vi "Script Add Constant VI --Project.vi"(4 "Project Ref":refnum<vi>, 6 "App Ref":refnum<vi>, 7 "Constant VI Name":string="TESTING.vi", 8 "error in":errorcluster, 9 "Constant VI Args":refnum<vi>) -> (0 "error out":errorcluster, 3 "Constant VI Path":path)   [LabVIEW 2020, in "ConstantErrorsMaker.lvlib"]
uses:
  ConstantErrorsMaker.lvlib
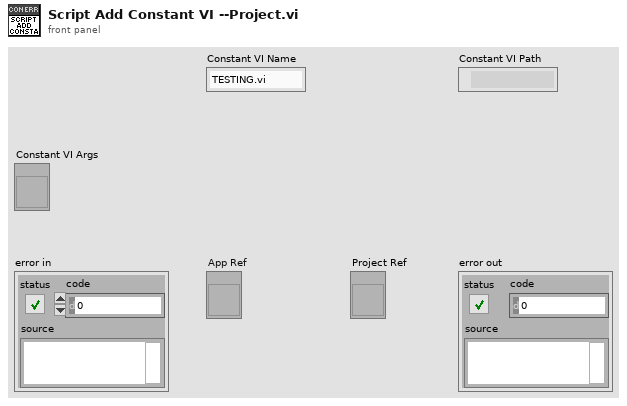
[diagram p1: front panel]
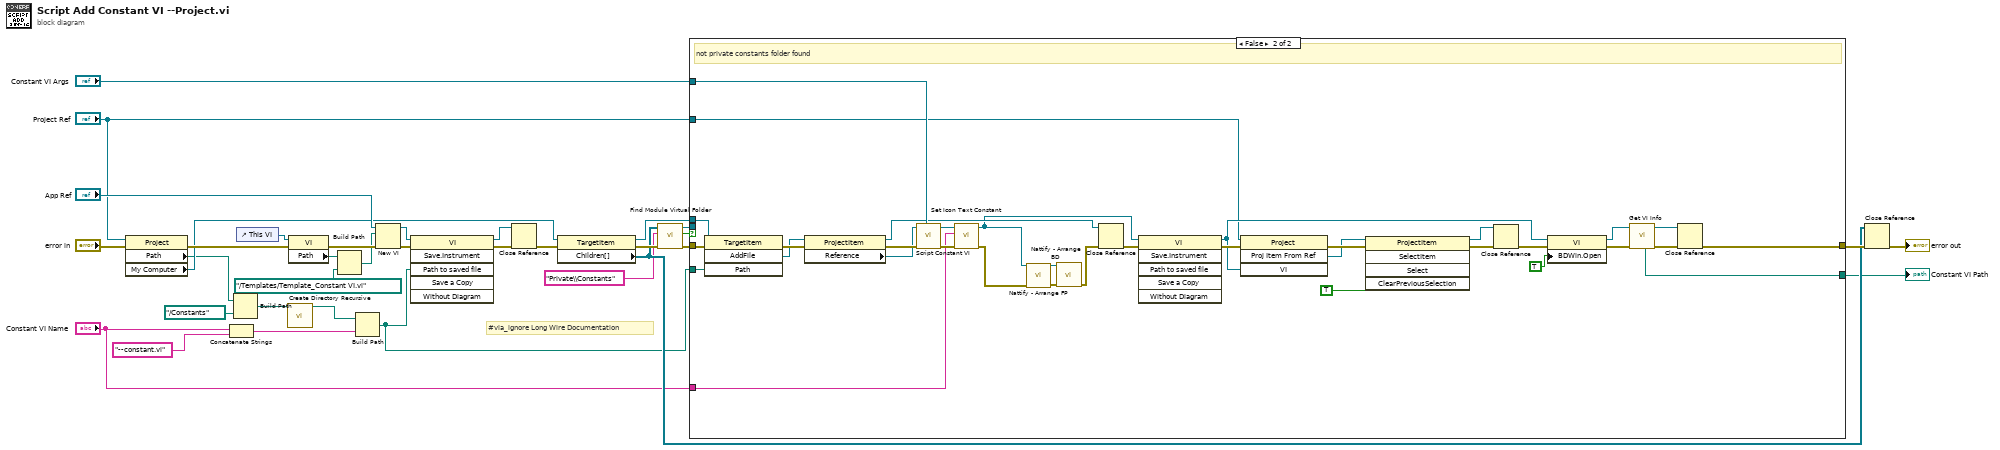
[diagram p0: block diagram]
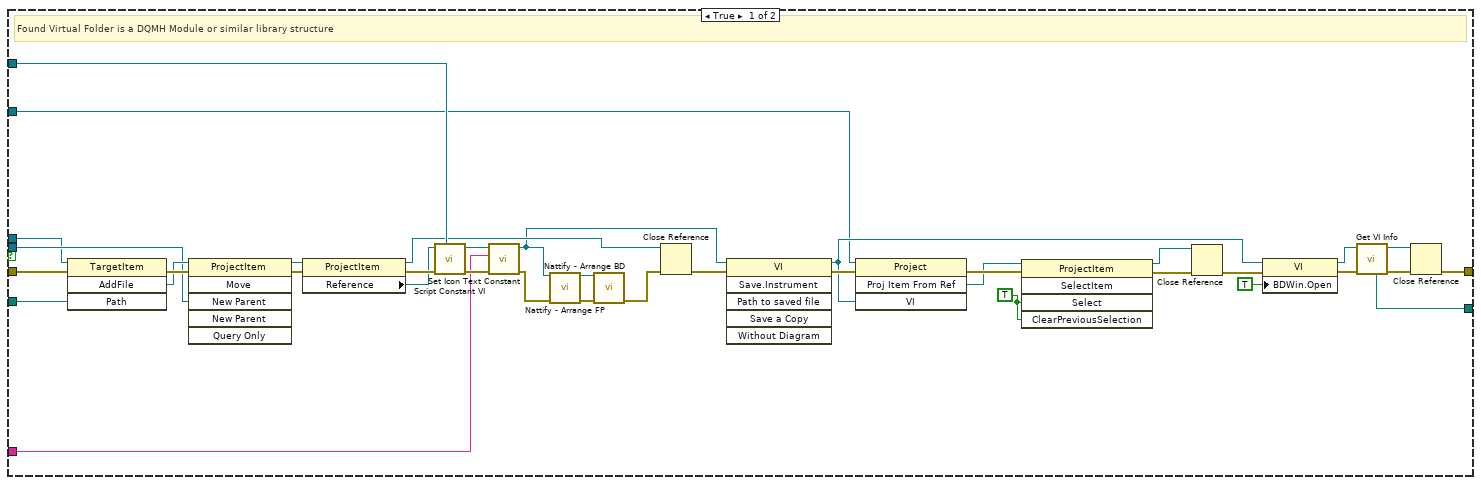
[diagram p2: hidden frame]
diagram:
  # "#via_ignore Long Wire Documentation"
  n1 = property class="Project"(reference="Project Ref", error in="error in") -> (error out=w31:errorcluster, "Path"=w4:path, "My Computer"=w5:refnum<vi>)  [unwired: 1 out]
  n2 = Concatenate Strings("Constant VI Name", "--constant.vi" ("input 1")) -> (w16:string)
  n3 = Build Path(base path=w4, name or relative path=path "../Constants") -> (appended path=w3:path)
  n4 = control-ref of="This VI"() -> (w15:refnum<vi>)
  n5 = call <vilib>:"Create Directory Recursive.vi"("directory"=w3) -> ("directory copy"=w1:path)  [unwired: 4 in, 2 out]
  n6 = property class="VI"(reference=w15, error in=w31) -> (error out=w25:errorcluster, "Path"=w14:path)  [unwired: 1 out]
  n7 = Build Path(base path=w14, name or relative path=path "../Templates/Template_Constant VI.vi") -> (appended path=w13:path)
  n8 = Build Path(base path=w1, name or relative path=w16) -> (appended path=w17:path)
  n9 = New VI(8:w25, 10:w13, 11:"App Ref") -> (0:w28:errorcluster, 3:w19:refnum<vi>)  [unwired: 4 in]
  n10 = invoke class="VI" method="Save.Instrument"(reference=w19, error in=w28, "Path to saved file"=w17) -> (reference out=w11:refnum<vi>, error out=w26:errorcluster)  [unwired: 3 in, 4 out]
  n11 = Close Reference(reference=w11, error in (no error)=w26) -> (error out=w27:errorcluster)
  n12 = property class="TargetItem"(reference=w5, error in=w27) -> (reference out=w6:refnum<vi>, error out=w33:errorcluster, "Children[]"=w22:refnum<vi>[])
  n13 = call "Find Module Virtual Folder.vi"("error in"=w33, "Virtual Folder"="Private\\Constants", "Children"=w22) -> ("error out"=w32:errorcluster, "Found?"=w23:bool, "ProjectItem out"=w24:refnum<vi>)  [unwired: 6 in]
  n14 = case shown="False" w23 {
    tunnel: [w63 w97] -> w34
    tunnel: w32 -> [w71 w105]
    tunnel: w24 -> [w54 _]
    tunnel: "Constant VI Args" -> [w52 w88]
    tunnel: w17 -> [w53 w89]
    tunnel: "Constant VI Name" -> [w45 w82]
    tunnel: "Project Ref" -> [w40 w78]
    tunnel: [w36 w73] -> w8
    tunnel: w6 -> [w35 w72]
    frame True {
      w43 = TRUE ("Select")
      # "Found Virtual Folder is a DQMH Module or similar library structure"
      n15 = invoke class="TargetItem" method="AddFile"(reference=w35, error in=w71, "Path"=w53) -> (error out=w70:errorcluster, "AddFile"=w55:refnum<vi>)  [unwired: 1 in, 2 out]
      n16 = invoke class="ProjectItem" method="Move"(reference=w55, error in=w70, "New Parent"=w54) -> (reference out=w50:refnum<vi>, error out=w69:errorcluster)  [unwired: 3 in, 4 out]
      n17 = property class="ProjectItem"(reference=w50, error in=w69) -> (reference out=w49:refnum<vi>, error out=w58:errorcluster, "Reference"=w39:refnum<vi>)
      n18 = call "Script Constant VI.vi"("Custom Argument Window"=w52, "error in"=w58, "VI Reference"=w39) -> ("error out"=w68:errorcluster, "VI reference"=w51:refnum<vi>)  [unwired: 7 in]
      n19 = call "Set Icon Text Constant.vi"("error in"=w68, "Text"=w45, "VI in"=w51) -> ("error out"=w66:errorcluster, "VI out"=w47:refnum<vi>)  [unwired: 7 in]
      n20 = call "Nattify - Arrange FP.vi"("VI in"=w47, "error in"=w66) -> ("VI out"=w48:refnum<vi>, "error out"=w67:errorcluster)  [unwired: 12 in]
      n21 = call "Nattify - Arrange BD.vi"("VI in"=w48, "error in"=w67) -> ("error out"=w64:errorcluster)  [unwired: 13 in]
      n22 = Close Reference(reference=w49, error in (no error)=w64) -> (error out=w56:errorcluster)
      n23 = invoke class="VI" method="Save.Instrument"(reference=w47, error in=w56) -> (reference out=w42:refnum<vi>, error out=w61:errorcluster)  [unwired: 4 in, 4 out]
      n24 = invoke class="Project" method="Proj Item From Ref"(reference=w40, error in=w61, "VI"=w42) -> (error out=w62:errorcluster, "ProjItemFromRef"=w44:refnum<vi>)  [unwired: 1 in, 2 out]
      n25 = invoke class="ProjectItem" method="SelectItem"(reference=w44, error in=w62, "Select"=w43, "ClearPreviousSelection"=w43) -> (reference out=w41:refnum<vi>, error out=w60:errorcluster)  [unwired: 1 in, 3 out]
      n26 = Close Reference(reference=w41, error in (no error)=w60) -> (error out=w59:errorcluster)
      n27 = property class="VI"(reference=w42, error in=w59, "BDWin.Open"=TRUE ("Block Diagram Window:Open")) -> (reference out=w38:refnum<vi>, error out=w65:errorcluster)
      n28 = call "Get VI Info.vi"("error in"=w65, "VI in"=w38) -> ("error out"=w57:errorcluster, "VI out"=w37:refnum<vi>, "VI Path"=w36:path)  [unwired: 4 in, 3 out]
      n29 = Close Reference(reference=w37, error in (no error)=w57) -> (error out=w63:errorcluster)
    }
    frame False {
      w80 = TRUE ("Select")
      # "not private constants folder found"
      n30 = invoke class="TargetItem" method="AddFile"(reference=w72, error in=w105, "Path"=w89) -> (error out=w96:errorcluster, "AddFile"=w90:refnum<vi>)  [unwired: 1 in, 2 out]
      n31 = property class="ProjectItem"(reference=w90, error in=w96) -> (reference out=w86:refnum<vi>, error out=w102:errorcluster, "Reference"=w76:refnum<vi>)
      n32 = call "Script Constant VI.vi"("Custom Argument Window"=w88, "error in"=w102, "VI Reference"=w76) -> ("error out"=w103:errorcluster, "VI reference"=w87:refnum<vi>)  [unwired: 7 in]
      n33 = call "Set Icon Text Constant.vi"("error in"=w103, "Text"=w82, "VI in"=w87) -> ("error out"=w100:errorcluster, "VI out"=w84:refnum<vi>)  [unwired: 7 in]
      n34 = call "Nattify - Arrange FP.vi"("VI in"=w84, "error in"=w100) -> ("VI out"=w85:refnum<vi>, "error out"=w101:errorcluster)  [unwired: 12 in]
      n35 = call "Nattify - Arrange BD.vi"("VI in"=w85, "error in"=w101) -> ("error out"=w98:errorcluster)  [unwired: 13 in]
      n36 = Close Reference(reference=w86, error in (no error)=w98) -> (error out=w104:errorcluster)
      n37 = invoke class="VI" method="Save.Instrument"(reference=w84, error in=w104) -> (reference out=w79:refnum<vi>, error out=w94:errorcluster)  [unwired: 4 in, 4 out]
      n38 = invoke class="Project" method="Proj Item From Ref"(reference=w78, error in=w94, "VI"=w79) -> (error out=w95:errorcluster, "ProjItemFromRef"=w81:refnum<vi>)  [unwired: 1 in, 2 out]
      n39 = invoke class="ProjectItem" method="SelectItem"(reference=w81, error in=w95, "Select"=w80, "ClearPreviousSelection"=w80) -> (reference out=w77:refnum<vi>, error out=w93:errorcluster)  [unwired: 1 in, 3 out]
      n40 = Close Reference(reference=w77, error in (no error)=w93) -> (error out=w92:errorcluster)
      n41 = property class="VI"(reference=w79, error in=w92, "BDWin.Open"=TRUE ("Block Diagram Window:Open")) -> (reference out=w75:refnum<vi>, error out=w99:errorcluster)
      n42 = call "Get VI Info.vi"("error in"=w99, "VI in"=w75) -> ("error out"=w91:errorcluster, "VI out"=w74:refnum<vi>, "VI Path"=w73:path)  [unwired: 4 in, 3 out]
      n43 = Close Reference(reference=w74, error in (no error)=w91) -> (error out=w97:errorcluster)
    }
  }
  "Constant VI Path" <- w8
  n44 = Close Reference(reference=w22, error in (no error)=w34) -> (error out=→"error out":errorcluster)
